vi "Define Enum Column.vi"(5 "Read Only":bool, 8 "Enum Reference":refnum<vi>, 9 "Tooltip":string, 10 "Caption":string, 11 "Name":string) -> (2 "Table Manager.lvlib:Column.lvclass:Column Descriptor":T1={"name"="Link", "caption"="", "Column Type"=enum."String", "Params"="", "AutoSizeMode"=1, "FillWeight"=100.0, "MinWidth"=50, "tooltip"="The quick brown fox jumps over the lazy dog", "Enum Reference"=refnum, "Channel suffix"="", "Read Only"=FALSE, "Call Back VI"=refnum, "DT Dependency"=0, "name dependency"=0, "data type"=enum."Double"} {"MinWidth" min=2 step=1; "AutoSizeMode" items=["None"=1, "ColumnHeader"=2, "AllCellsExceptHeader"=4, "AllCells"=6, "DisplayedCellsExceptHeader"=8, "DisplayedCells"=10, "Fill"=16]; "FillWeight" min=1 max=100})   [LabVIEW 2013]
doc: "This VI describes a Mapping column that will map a channel to a tag. \nTHe name of the channel is built concatenating the name dependecy column value with the channel suffix. The datatype will be the value of the column indicated in DT dependecy if its (-1) it will use the Datatype control"
uses:
  Column/Column Descriptor.ctl
  Column/Column Type.ctl
  <vilib>/NI/Tag Bus/tag/Data Type.ctl
  Table Manager/Call Back Ref Type Def.ctl
  <vilib>/NI/DCAF/Tag Editor Core/Configuration Editor/Classes/Engine Parent/Engine Parent Editor Node.lvclass
  <vilib>/NI/DCAF/Tag Editor Core/Configuration Editor/Classes/Module editor node/module editor node.lvclass
  Column/Column.lvclass
  <vilib>/NI/Tag Bus/tag/tag descriptor.lvclass
  Table Manager/Table Manager.lvclass
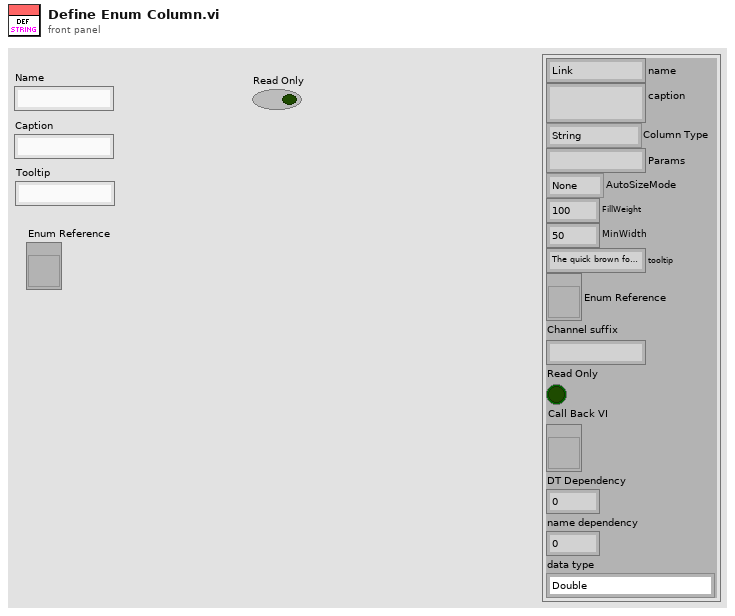
[diagram p1: front panel]
types:
  T1 = typedef "Table Manager.lvlib/Column.lvclass/Column Descriptor.ctl" = cluster{"name":string, "caption":string, "Column Type":T2, "Params":string, "AutoSizeMode":i32, "FillWeight":sgl, "MinWidth":u32, "tooltip":string, "Enum Reference":refnum<vi>, "Channel suffix":string, "Read Only":bool, "Call Back VI":T3, "DT Dependency":i32, "name dependency":i32, "data type":T4}
  T2 = typedef "Table Manager.lvlib/Column.lvclass/Column Type.ctl" = enum16{"String", "Mapping", "Channel Name", "Tag", "Enum", "Data Type", "Numeric"}
  T3 = typedef "Table Manager.lvlib/Table Manager.lvclass/Call Back Ref Type Def.ctl" = refnum<vi>
  T4 = typedef "tag bus.lvlib/tag descriptor.lvclass/Data Type.ctl" = enum16{"Double", "Single", "I64", "I32", "I16", "I8", "U64", "U32", "U16", "U8", "Boolean", "String", "Array of Double", "Array of Single", "Array of I64", "Array of I32", "Array of I16", "Array of I8", "Array of U64", "Array of U32", "Array of U16", "Array of U8", "Array of Boolean", "Array of String"}
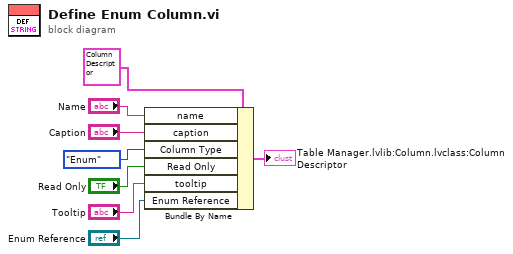
[diagram p0: block diagram]
diagram:
  n1 = Bundle By Name(cluster=T1 {"name"="", "caption"="", "Column Type"=enum."String", "Params"="", "AutoSizeMode"=16, "FillWeight"=100.0, "MinWidth"=50, "tooltip"="", "Enum Reference"=refnum, "Channel suffix"="", "Read Only"=FALSE, "Call Back VI"=refnum, "DT Dependency"=0, "name dependency"=0, "data type"=enum."Double"} ("Table Manager.lvlib:Column.lvclass:Column Descriptor"), "name"="Name", "caption"="Caption", "Column Type"=Column_Type."Enum", "Read Only"="Read Only", "tooltip"="Tooltip", "Enum Reference"="Enum Reference") -> (→"Table Manager.lvlib:Column.lvclass:Column Descriptor":T1)
